vi "DriveTest.vi"() -> ()   [LabVIEW 2018]
panel:
  in  "VasenSpeed 2":dbl
  out "CM Vasen 2":dbl
  out "CM Oikea 2":dbl
  in  "OikeaSpeed 2":dbl
  in  "EtuSpeed 2":dbl
  out "CM Etu 2":dbl
  in  "TakaSpeed 2":dbl
  out "CM Taka 2":dbl
  out "CM Taka":dbl
  in  "TakaSpeed":dbl
  out "CM Etu":dbl
  in  "EtuSpeed":dbl
  in  "OikeaSpeed":dbl
  out "CM Oikea":dbl
  out "CM Vasen":dbl
  in  "VasenSpeed":dbl
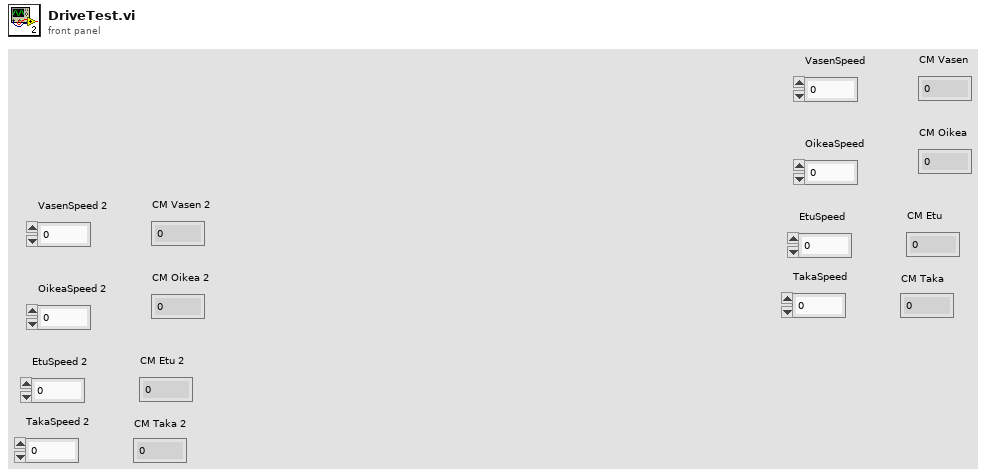
[diagram p1: front panel]
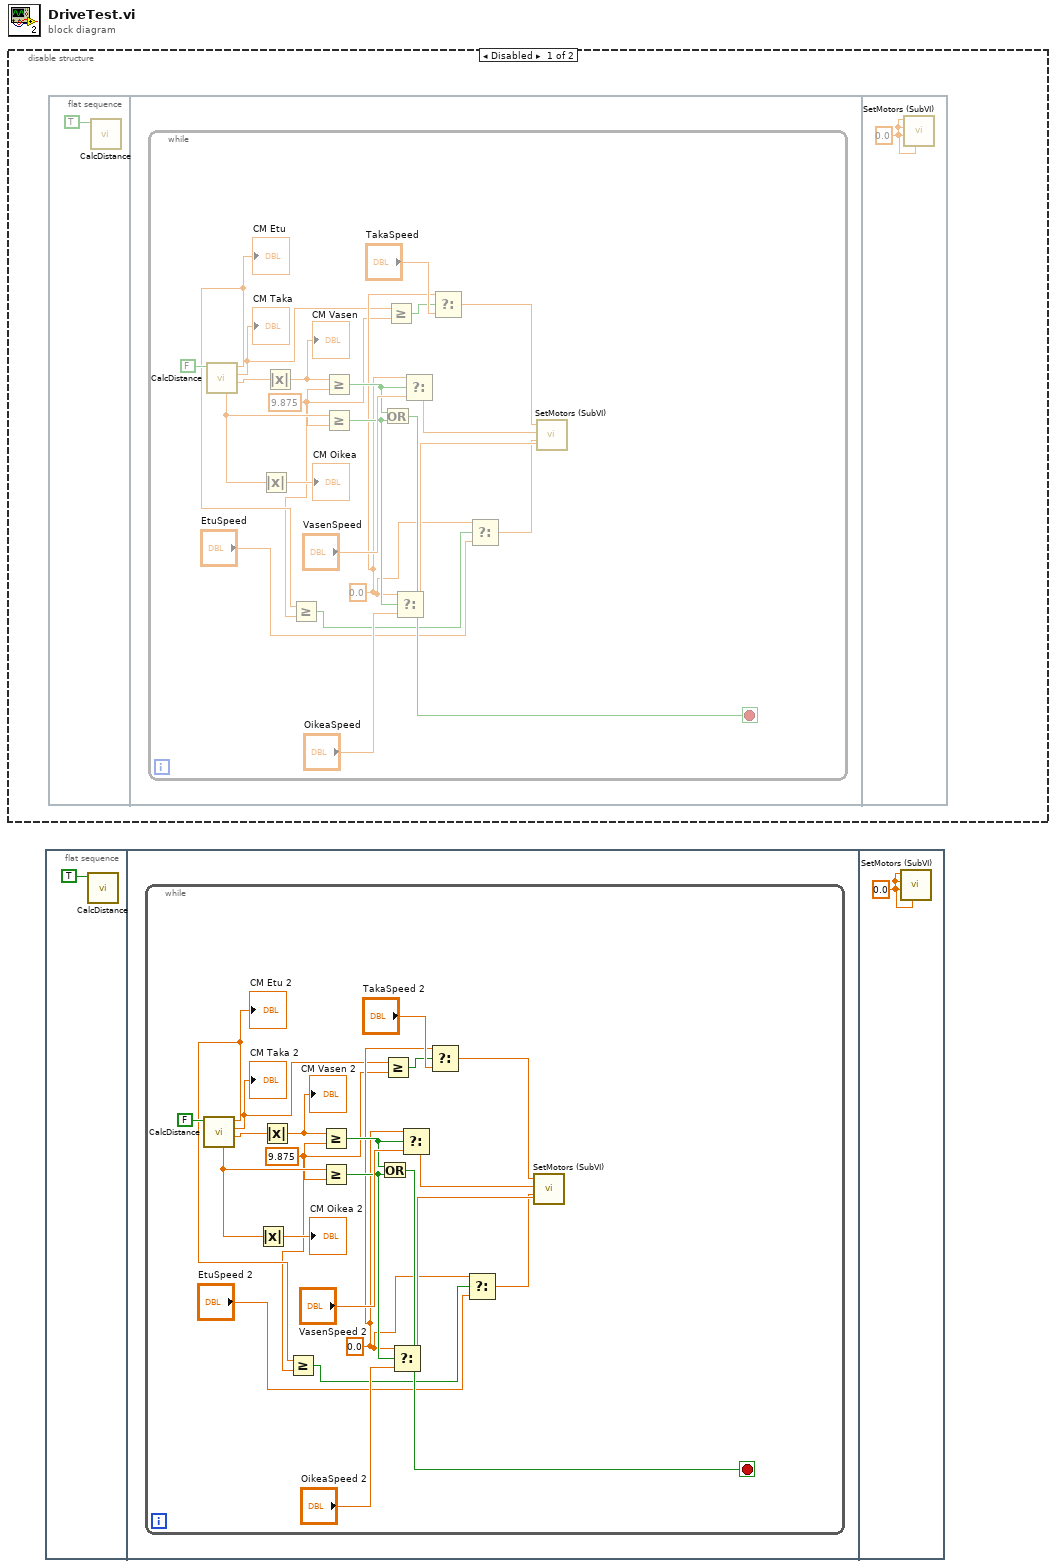
[diagram p0: block diagram]
diagram:
  n1 = disable-structure shown="Disabled" {
    frame Disabled {
      n2 = flat-sequence {
        frame #0 {
          n3 = call "CalcDistance.vi"("Reset Encoders"=TRUE) -> ()  [unwired: 7 in, 4 out]
        }
        frame #1 {
          n4 = while {
            stop <- w20 stop-if-true
            w9 = 0.0 ("t")
            w5 = 9.875 ("t")
            n5 = call "CalcDistance.vi"("Reset Encoders"=FALSE) -> ("CM Vasen"=w17:dbl, "CM Taka"=w7:dbl, "CM Etu"=w6:dbl, "CM Oikea"=w13:dbl)  [unwired: 7 in]
            "CM Etu" <- w6
            "CM Taka" <- w7
            n6 = Absolute Value(x=w13) -> (abs(x)=→"CM Oikea":dbl)
            n7 = Absolute Value(x=w17) -> (abs(x)=w18:dbl)
            "CM Vasen" <- w18
            n8 = Greater Or Equal?(x=w6, y=w5) -> (x >= y?=w2:bool)
            n9 = Greater Or Equal?(x=w18, y=w5) -> (x >= y?=w19:bool)
            n10 = Greater Or Equal?(x=w13, y=w5) -> (x >= y?=w16:bool)
            n11 = Or(x=w19, y=w16) -> (x .or. y?=w20:bool)
            n12 = Greater Or Equal?(x=w7, y=w5) -> (x >= y?=w8:bool)
            n13 = Select(t=w9, s=w16, f="OikeaSpeed") -> (s? t:f=w14:dbl)
            n14 = Select(t=w9, s=w19, f="VasenSpeed") -> (s? t:f=w21:dbl)
            n15 = Select(t=w9, s=w8, f="TakaSpeed") -> (s? t:f=w3:dbl)
            n16 = Select(t=w9, s=w2, f="EtuSpeed") -> (s? t:f=w4:dbl)
            n17 = call "SetMotors (SubVI).vi"("Oikea"=w14, "Etu"=w4, "Vasen"=w21, "Taka"=w3) -> ()  [unwired: 8 in]
          }
        }
        frame #2 {
          w24 = 0.0 ("Taka")
          n18 = call "SetMotors (SubVI).vi"("Oikea"=w24, "Etu"=w24, "Vasen"=w24, "Taka"=w24) -> ()  [unwired: 8 in]
        }
      }
    }
    frame Enabled {
    }
  }
  n19 = flat-sequence {
    frame #0 {
      n20 = call "CalcDistance.vi"("Reset Encoders"=TRUE) -> ()  [unwired: 7 in, 4 out]
    }
    frame #1 {
      n21 = while {
        stop <- w44 stop-if-true
        w33 = 0.0 ("t")
        w29 = 9.875 ("t")
        n22 = call "CalcDistance.vi"("Reset Encoders"=FALSE) -> ("CM Vasen"=w41:dbl, "CM Taka"=w31:dbl, "CM Etu"=w30:dbl, "CM Oikea"=w37:dbl)  [unwired: 7 in]
        "CM Etu 2" <- w30
        "CM Taka 2" <- w31
        n23 = Absolute Value(x=w37) -> (abs(x)=→"CM Oikea 2":dbl)
        n24 = Absolute Value(x=w41) -> (abs(x)=w42:dbl)
        "CM Vasen 2" <- w42
        n25 = Greater Or Equal?(x=w30, y=w29) -> (x >= y?=w26:bool)
        n26 = Greater Or Equal?(x=w42, y=w29) -> (x >= y?=w43:bool)
        n27 = Greater Or Equal?(x=w37, y=w29) -> (x >= y?=w40:bool)
        n28 = Or(x=w43, y=w40) -> (x .or. y?=w44:bool)
        n29 = Greater Or Equal?(x=w31, y=w29) -> (x >= y?=w32:bool)
        n30 = Select(t=w33, s=w40, f="OikeaSpeed 2") -> (s? t:f=w38:dbl)
        n31 = Select(t=w33, s=w43, f="VasenSpeed 2") -> (s? t:f=w45:dbl)
        n32 = Select(t=w33, s=w32, f="TakaSpeed 2") -> (s? t:f=w27:dbl)
        n33 = Select(t=w33, s=w26, f="EtuSpeed 2") -> (s? t:f=w28:dbl)
        n34 = call "SetMotors (SubVI).vi"("Oikea"=w38, "Etu"=w28, "Vasen"=w45, "Taka"=w27) -> ()  [unwired: 8 in]
      }
    }
    frame #2 {
      w48 = 0.0 ("Taka")
      n35 = call "SetMotors (SubVI).vi"("Oikea"=w48, "Etu"=w48, "Vasen"=w48, "Taka"=w48) -> ()  [unwired: 8 in]
    }
  }
